vi "Make Protection Signal.vi"(11 "Node Ptr":T1=18446744073709551615 format="%.0x") -> ()   [LabVIEW 2015, in "J1939 Addon System Explorer.lvlib"]
uses:
  J1939 Addon System Explorer.lvlib
  <vilib>/NI Veristand/Custom Device API/Custom Device Item Ref.ctl
  Shared/SubVIs/Constants.vi
  Shared/J1939 Addon Shared.lvlib
  SubModules/Frame Protection Support/Source/System Explorer/Protection and Counter Support System Explorer.lvlib
  <vilib>/NI VeriStand/Custom Device API/Custom Device API.lvlib
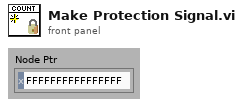
[diagram p1: front panel]
types:
  T1 = typedef "Custom Device API.lvlib/Custom Device Item Ref.ctl" = u64
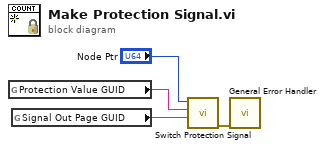
[diagram p0: block diagram]
diagram:
  n1 = global read "Constants.vi" "Protection Value GUID"() -> (w2:string)
  n2 = global read "Constants.vi" "Signal Out Page GUID"() -> (w3:string)
  n3 = call "Switch Protection Signal.vi"("Signal Page GUID"=w3, "Protection Value GUID"=w2, "Node Ptr"="Node Ptr") -> ("error out"=w4:errorcluster)  [unwired: 8 in]
  n4 = call <vilib>:"General Error Handler.vi"("error in (no error)"=w4) -> ()  [unwired: 10 in, 5 out]
